vi "Config_Instrument.vi"() -> ()   [LabVIEW 2015]
uses:
  Program Files/National Instruments/LabVIEW 2015/examples/Instrument IO/Serial/support/Serial - Settings.ctl
  <vilib>/Instr/_visa.llb/VISA Configure Serial Port (Instr).vi
  Global_Serial.vi
  <instrlib>/Agilent E363X Series/Agilent E363X Series.lvlib
  <instrlib>/Rohde&Schwarz Spectrum Analyzer/Rohde&Schwarz Spectrum Analyzer.lvlib
panel:
  out "R&S Spec2":refnum<visa-resource-name>
  out "R&S Spec1":refnum<visa-resource-name>
  out "LED_K6":bool
  in  "OK":bool=TRUE
  out "LED_RSSMA":bool
  out "LED_K4":bool
  out "LED_RS S2":bool
  in  "RBW2(HZ)":dbl(knob)=2100000000.0 scale=1000000.0..8000000000.0 scale format="%#_4p"
  in  "Stop Frequency2 (Hz)":dbl(knob)=2100000000.0 scale=1000000.0..8000000000.0 scale format="%#_4p"
  in  "Start Frequency2 (Hz)":dbl(knob)=2100000000.0 scale=1000000.0..8000000000.0 scale format="%#_4p"
  out "LED_RS S1":bool
  in  "RBW(HZ)":dbl(knob)=2100000000.0 scale=1000000.0..8000000000.0 scale format="%#_4p"
  in  "Stop Frequency (Hz)":dbl(knob)=2100000000.0 scale=1000000.0..8000000000.0 scale format="%#_4p"
  in  "Start Frequency (Hz)":dbl(knob)=2100000000.0 scale=1000000.0..8000000000.0 scale format="%#_4p"
  in  "Open XXXXXXXXXXXX":bool
  in  "Open R&S SMA200":bool
  in  "Open R&S Spectrum2":bool
  in  "Open R&S Spectrum1":bool
  in  "Open R&S SMA100":bool
  in  "Open KEYSIGHE E3631#4":bool
  in  "Open KEYSIGHE E3631#6":bool
  in  "SPAN2":dbl(slide)=1000000000.0 scale=1000000.0..8000000000.0 scale format="%#.2p"
  in  "OFFSET2(dBm)":dbl(slide) scale=-20.0..30.0 scale format="%#.2f"
  in  "REF LEVEL2(dBm)":dbl(slide) scale=-20.0..30.0 scale format="%#.2f"
  in  "Center Frequency2(Hz)":dbl(knob)=2100000000.0 scale=1000000.0..8000000000.0 scale format="%#_4p"
  in  "R&S Spectrum2":refnum<visa-resource-name>="COM1"
  in  "SPAN":dbl(slide)=1000000000.0 scale=1000000.0..8000000000.0 scale format="%#.2p"
  in  "OFFSET(dBm)":dbl(slide) scale=-20.0..30.0 scale format="%#.2f"
  in  "REF LEVEL(dBm)":dbl(slide) scale=-20.0..30.0 scale format="%#.2f"
  in  "Center Frequency (Hz)":dbl(knob)=2100000000.0 scale=1000000.0..8000000000.0 scale format="%#_4p"
  in  "R&S Spectrum1":refnum<visa-resource-name>="COM1"
  in  "RF ON":bool
  in  "RF Level(dBm)":dbl(slide) scale=-146.0..18.0 scale format="%#.2f"
  in  "RF Phase":dbl(slide)=154517.79084245834 step=1.0 scale=-360.0..360.0 scale format="%#_6p"
  in  "RF Frequency (Hz)":dbl(knob)=205410.22592152198 scale=1000000.0..3000000000.0 scale format="%#_6p"
  in  "R&S SMA100":refnum<visa-resource-name>="COM1"
  in  "CH2#4":bool
  in  "CH3#4":bool
  in  "CH1#4":bool
  in  "CH2#6":bool
  in  "CH3#6":bool
  in  "CH1#6":bool
  in  "#4最小输入电压(V)":i32=1 min=0 max=6
  in  "#4最大输入电压(V)":i32=2 min=0 max=6
  in  "#6最小输入电压(V)":i32 min=0
  in  "#6最大输入电压(V)":i32=3 min=0
  in  "CC3#4(A)":dbl(slide) scale=0.0..1.0 scale format="%#.2f"
  in  "CC2#4(A)":dbl(slide) scale=0.0..1.0 scale format="%#.2f"
  in  "CC1#4(A)":dbl(slide) scale=0.0..5.0 scale format="%#.2f"
  in  "CV2#4(V)":dbl(slide) scale format="%#.2f"
  in  "CV1#4(V)":dbl(slide) scale=0.0..25.0 scale format="%#.2f"
  in  "CV3#4(V)":dbl(slide) scale=0.0..6.0 scale format="%#.2f"
  out "Instrument Driver Revision 2":string="*IDN?"
  in  "CC3#6(A)":dbl(slide) scale=0.0..1.0 scale format="%#.2f"
  in  "CC2#6(A)":dbl(slide) scale=0.0..1.0 scale format="%#.2f"
  in  "CC1#6(A)":dbl(slide) scale=0.0..5.0 scale format="%#.2f"
  in  "CV2#6(V)":dbl(slide) scale format="%#.2f"
  in  "CV1#6(V)":dbl(slide) scale=0.0..25.0 scale format="%#.2f"
  in  "CV3#6(V)":dbl(slide) scale=0.0..6.0 scale format="%#.2f"
  out "Instrument Driver Revision":string="*IDN?"
  in  "KeysightE363x_#4":refnum<visa-resource-name>="COM1"
  in  "KeysightE363x_#6":refnum<visa-resource-name>="COM1"
  in  "stop":bool
  in  "error in (no error)":errorcluster
  in  "SerialON":bool
  in  "Serial Settings":T1={"baud rate"=9600, "data bits"=8, "parity"=enum."None", "stop bits"=10, "flow control"=0} {"flow control" items=["None"=0, "XON/XOFF"=1, "RTS/CTS"=2, "DTR/DSR"=4]; "stop bits" items=["1.0"=10, "1.5"=15, "2.0"=20]; "data bits" min=5 max=8 step=1; "baud rate" items=["75"=75, "110"=110, "134"=134, "150"=150, "300"=300, "600"=600, "1200"=1200, "1800"=1800, "2400"=2400, "4800"=4800, "7200"=7200, "9600"=9600, "14400"=14400, "19200"=19200, "28800"=28800, "38400"=38400, "56000"=56000, "57600"=57600, "115200"=115200, "128000"=128000, "230400"=230400]}
  in  "Serial Port":refnum<visa-resource-name>="COM1"
  # "缺省信号源"
  # "缺省信号源"
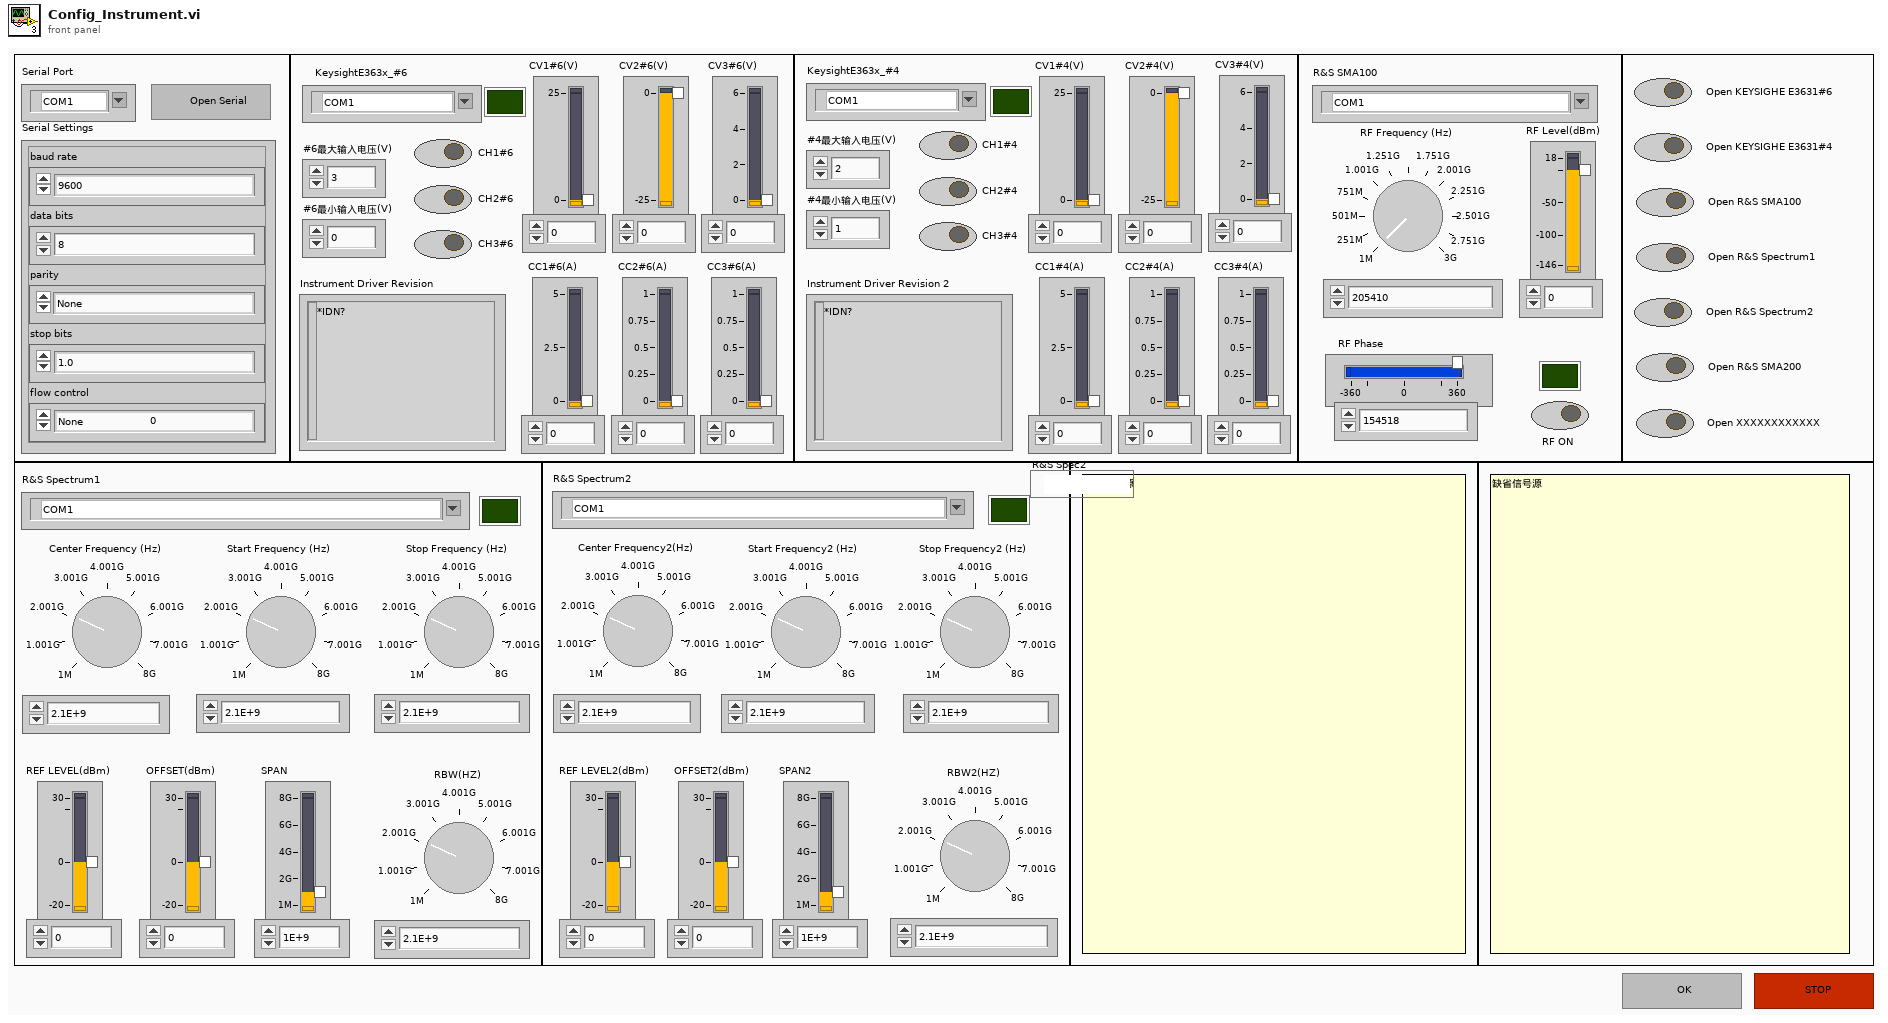
[diagram p1: front panel]
types:
  T1 = typedef "Serial - Settings.ctl" = cluster{"baud rate":u32, "data bits":u16, "parity":enum16{"None", "Odd", "Even", "Mark", "Space"}, "stop bits":u16, "flow control":u16}
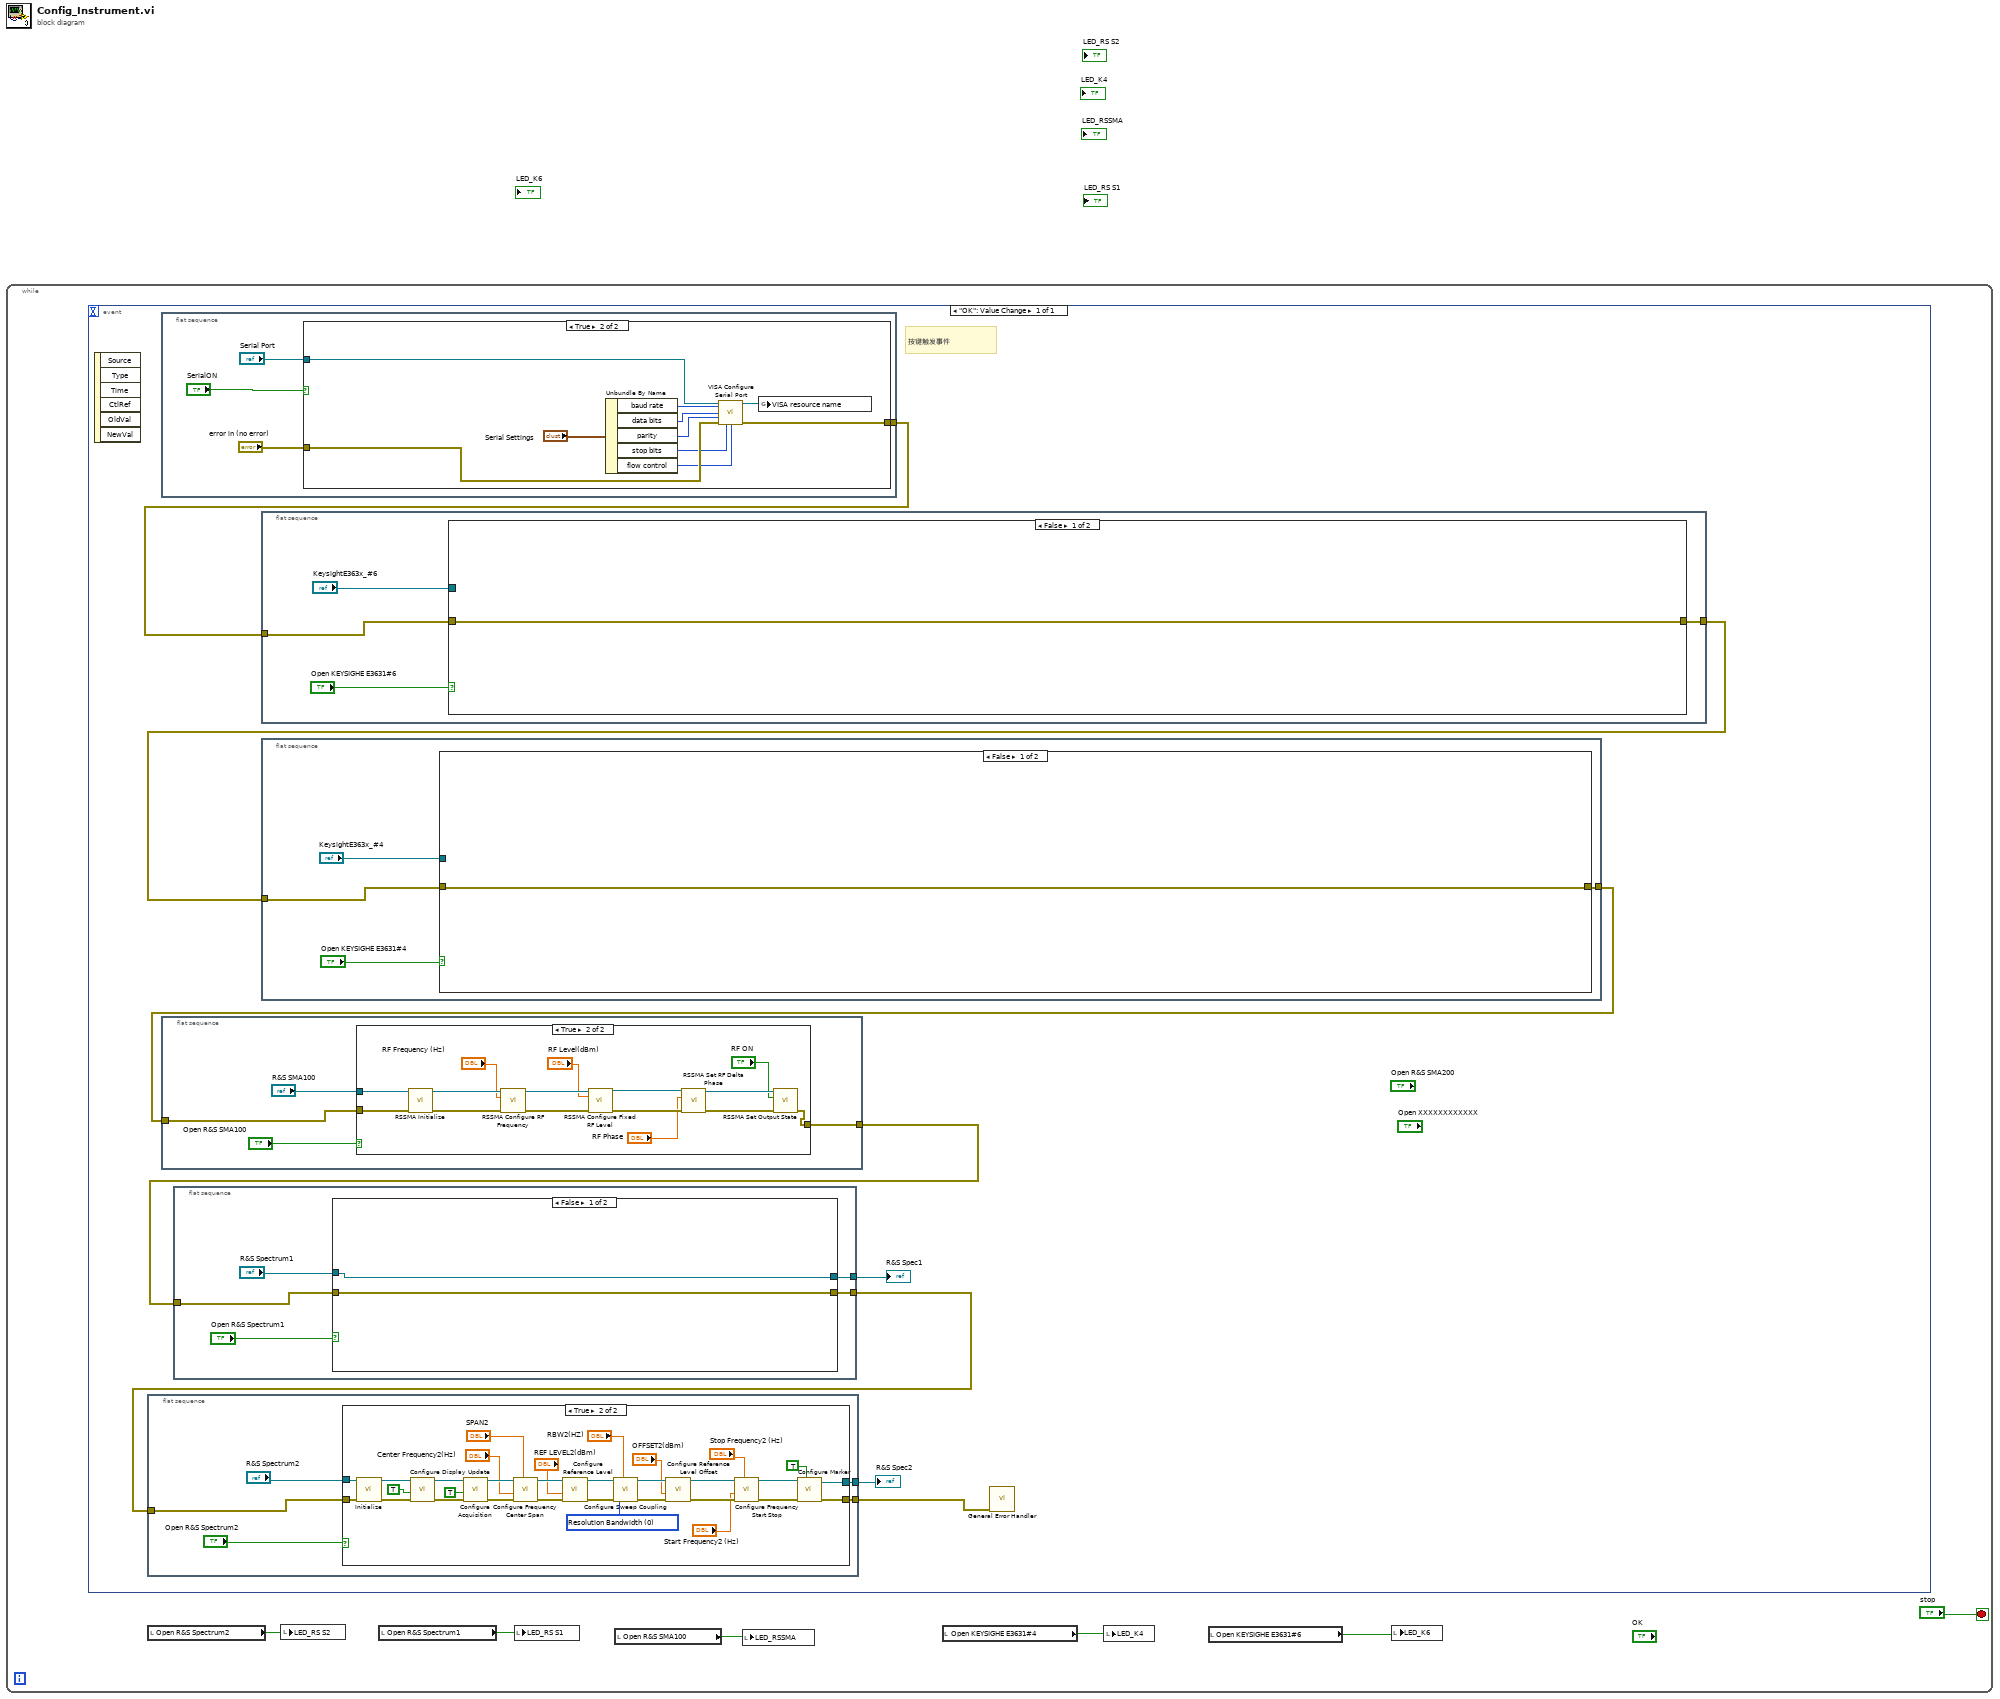
[diagram p0: block diagram]
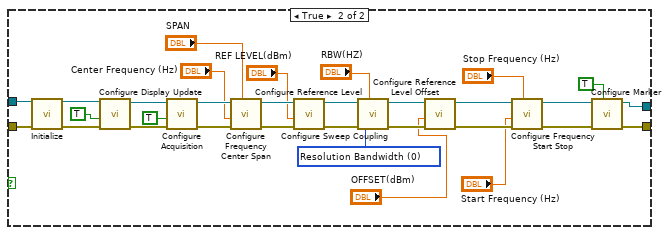
[diagram p3: hidden frame]
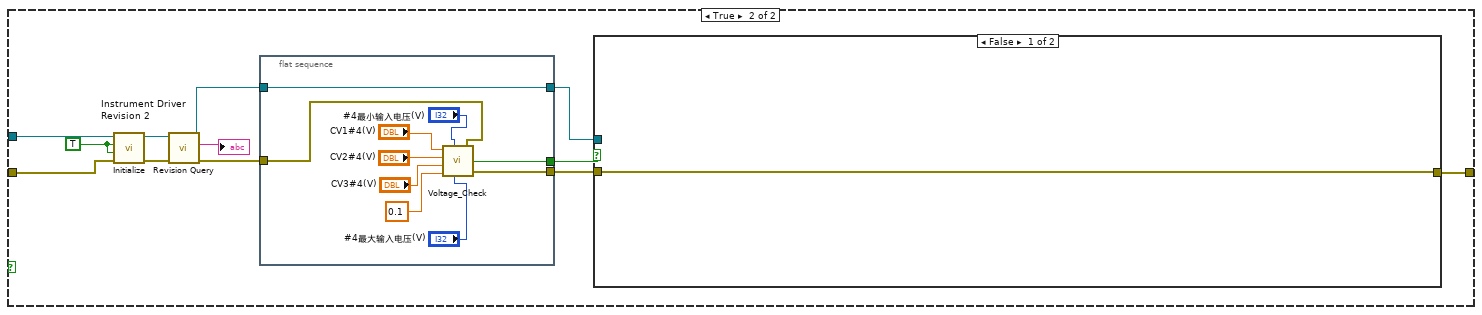
[diagram p5: hidden frame]
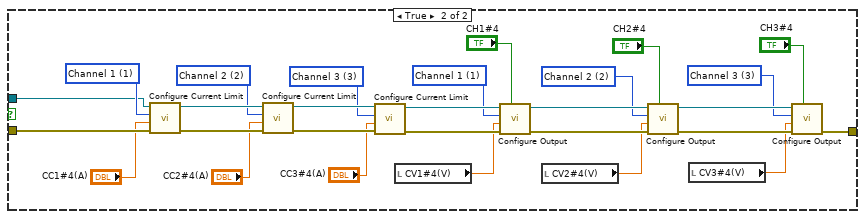
[diagram p6: hidden frame]
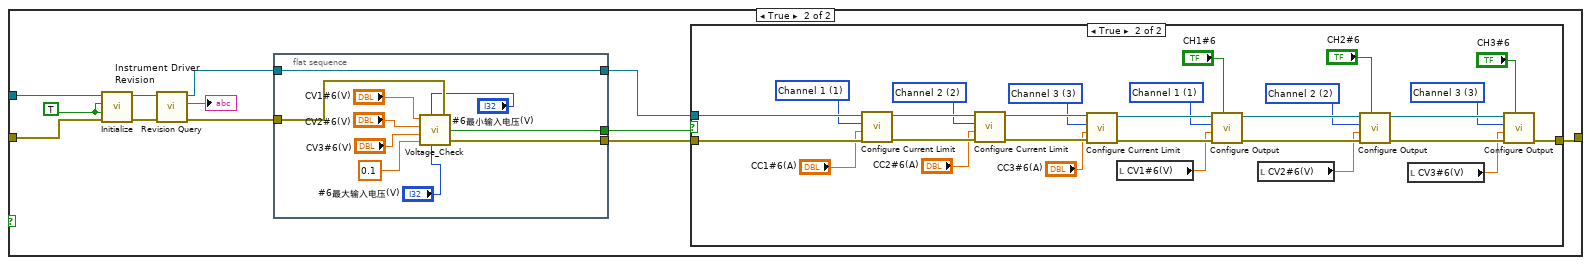
[diagram p7: hidden frame]
diagram:
  n1 = while {
    stop <- "stop" stop-if-true
    n2 = event shown="[0] \"OK\": Value Change" {
      selector: _ -> [_]
      dyn-events: _ -> [_]
      timeout: _ -> [_]
      event "OK": Value Change {
        # "按键触发事件"
        n3 = event-data() -> ()  [unwired: 1 in, 6 out]
        n4 = flat-sequence {
          tunnel: w10 -> [w17]
          tunnel: [w16] -> w9
          tunnel: [w15] -> w7
          frame #0 {
            n5 = case shown="True" "Open R&S Spectrum2" {
              tunnel: w17 -> [w21 w36]
              tunnel: "R&S Spectrum2" -> [w20 w27]
              tunnel: [w21 w23] -> w16
              tunnel: [w20 w22] -> w15
              frame False {
              }
              frame True {
                w37 = 0 items=["Resolution Bandwidth", "Video Bandwidth", "Sweep Time"] ("Sweep Coupling (Resolution Bandwidth)")
                n6 = call <instrlib>:"Initialize.vi"("VISA resource name"=w27, "error in (no error)"=w36) -> ("VISA resource name out"=w50:refnum<visa-resource-name>, "error out"=w51:errorcluster)  [unwired: 12 in]
                n7 = call <instrlib>:"Configure Display Update.vi"("error in (no error)"=w51, "Display In Remote (F: Off)"=TRUE, "VISA resource name"=w50) -> ("error out"=w49:errorcluster, "VISA resource name out"=w48:refnum<visa-resource-name>)  [unwired: 7 in]
                n8 = call <instrlib>:"Configure Acquisition.vi"("error in (no error)"=w49, "Sweep Mode Continuous (F: Off)"=TRUE, "VISA resource name"=w48) -> ("error out"=w46:errorcluster, "VISA resource name out"=w45:refnum<visa-resource-name>)  [unwired: 7 in]
                n9 = call <instrlib>:"Configure Frequency Center Span.vi"("Span (0.0)"="SPAN2", "error in (no error)"=w46, "Center Frequency (0.0)"="Center Frequency2(Hz)", "VISA resource name"=w45) -> ("error out"=w44:errorcluster, "VISA resource name out"=w43:refnum<visa-resource-name>)  [unwired: 6 in]
                n10 = call <instrlib>:"Configure Reference Level.vi"("error in (no error)"=w44, "Reference Level (-20.0)"="REF LEVEL2(dBm)", "VISA resource name"=w43) -> ("error out"=w42:errorcluster, "VISA resource name out"=w41:refnum<visa-resource-name>)  [unwired: 7 in]
                n11 = call <instrlib>:"Configure Sweep Coupling.vi"("Coupling Value (0.0)"="RBW2(HZ)", "error in (no error)"=w42, "Sweep Coupling (Resolution Bandwidth)"=w37, "VISA resource name"=w41) -> ("error out"=w40:errorcluster, "VISA resource name out"=w39:refnum<visa-resource-name>)  [unwired: 6 in]
                n12 = call <instrlib>:"Configure Reference Level Offset.vi"("error in (no error)"=w40, "Reference Level Offset (0.0)"="OFFSET2(dBm)", "VISA resource name"=w39) -> ("error out"=w35:errorcluster, "VISA resource name out"=w34:refnum<visa-resource-name>)  [unwired: 7 in]
                n13 = call <instrlib>:"Configure Frequency Start Stop.vi"("Stop Frequency (0.0)"="Stop Frequency2 (Hz)", "error in (no error)"=w35, "Start Frequency (0.0)"="Start Frequency2 (Hz)", "VISA resource name"=w34) -> ("error out"=w33:errorcluster, "VISA resource name out"=w32:refnum<visa-resource-name>)  [unwired: 6 in]
                n14 = call <instrlib>:"Configure Marker.vi"("Marker State (F: Off)"=TRUE, "error in (no error)"=w33, "VISA resource name"=w32) -> ("error out"=w23:errorcluster, "VISA resource name out"=w22:refnum<visa-resource-name>)  [unwired: 7 in]
              }
            }
          }
        }
        n15 = flat-sequence {
          tunnel: [w223] -> w14
          frame #0 {
            n16 = case shown="True" "SerialON" {
              tunnel: "Serial Port" -> [_ w237]
              tunnel: "error in (no error)" -> [w227 w236]
              tunnel: [w227 w229] -> w223
              frame False {
              }
              frame True {
                n17 = Unbundle By Name("Serial Settings") -> ("baud rate"=w231:u32, "data bits"=w232:u16, "parity"=w233:enum16{"None", "Odd", "Even", "Mark", "Space"}, "stop bits"=w234:u16, "flow control"=w235:u16)
                n18 = call-poly "VISA Configure Serial Port"("VISA resource name"=w237, "baud rate (9600)"=w231, "data bits (8)"=w232, "parity (0:none)"=w233, "error in (no error)"=w236, "stop bits (10: 1 bit)"=w234, "flow control (0:none)"=w235) -> ("VISA resource name out"=w228:refnum<visa-resource-name>, "error out"=w229:errorcluster)  [unwired: 7 in]
                n19 = global write "Global_Serial.vi" "VISA resource name"(w228) -> ()
              }
            }
          }
        }
        n20 = flat-sequence {
          tunnel: w12 -> [w92]
          tunnel: [w91] -> w11
          frame #0 {
            n21 = case shown="True" "Open R&S SMA100" {
              tunnel: "R&S SMA100" -> [_ w102]
              tunnel: w92 -> [w95 w101]
              tunnel: [w95 w96] -> w91
              frame False {
              }
              frame True {
                n22 = call <instrlib>:"RSSMA Initialize.vi"("error in (no error)"=w101, "Resource Name (GPIB::28)"=w102) -> ("error out"=w110:errorcluster, "dup VISA session"=w109:refnum<visa-resource-name>)  [unwired: 8 in]
                n23 = call <instrlib>:"RSSMA Configure RF Frequency.vi"("error in (no error)"=w110, "Frequency (1.0e9 Hz)"="RF Frequency (Hz)", "VISA session"=w109) -> ("error out"=w108:errorcluster, "dup VISA session"=w107:refnum<visa-resource-name>)  [unwired: 7 in]
                n24 = call <instrlib>:"RSSMA Configure Fixed RF Level.vi"("VISA session"=w107, "Amplitude (-30.0 dBm)"="RF Level(dBm)", "error in (no error)"=w108) -> ("dup VISA session"=w105:refnum<visa-resource-name>, "error out"=w106:errorcluster)  [unwired: 11 in]
                n25 = call <instrlib>:"RSSMA Set RF Delta Phase.vi"("error in (no error)"=w106, "Delta Phase (0.0)"="RF Phase", "VISA session"=w105) -> ("error out"=w104:errorcluster, "dup VISA session"=w103:refnum<visa-resource-name>)  [unwired: 7 in]
                n26 = call <instrlib>:"RSSMA Set Output State.vi"("error in (no error)"=w104, "RF Output State (F: Off)"="RF ON", "VISA session"=w103) -> ("error out"=w96:errorcluster)  [unwired: 7 in, 1 out]
              }
            }
          }
        }
        n27 = flat-sequence {
          tunnel: w11 -> [w55]
          tunnel: [w54] -> w10
          tunnel: [w53] -> w8
          frame #0 {
            n28 = case shown="False" "Open R&S Spectrum1" {
              tunnel: w55 -> [w59 w74]
              tunnel: "R&S Spectrum1" -> [w58 w69]
              tunnel: [w59 w61] -> w54
              tunnel: [w58 w60] -> w53
              frame False {
              }
              frame True {
                w75 = 0 items=["Resolution Bandwidth", "Video Bandwidth", "Sweep Time"] ("Sweep Coupling (Resolution Bandwidth)")
                n29 = call <instrlib>:"Initialize.vi"("VISA resource name"=w69, "error in (no error)"=w74) -> ("VISA resource name out"=w88:refnum<visa-resource-name>, "error out"=w89:errorcluster)  [unwired: 12 in]
                n30 = call <instrlib>:"Configure Display Update.vi"("error in (no error)"=w89, "Display In Remote (F: Off)"=TRUE, "VISA resource name"=w88) -> ("error out"=w87:errorcluster, "VISA resource name out"=w86:refnum<visa-resource-name>)  [unwired: 7 in]
                n31 = call <instrlib>:"Configure Acquisition.vi"("error in (no error)"=w87, "Sweep Mode Continuous (F: Off)"=TRUE, "VISA resource name"=w86) -> ("error out"=w84:errorcluster, "VISA resource name out"=w83:refnum<visa-resource-name>)  [unwired: 7 in]
                n32 = call <instrlib>:"Configure Frequency Center Span.vi"("Span (0.0)"="SPAN", "error in (no error)"=w84, "Center Frequency (0.0)"="Center Frequency (Hz)", "VISA resource name"=w83) -> ("error out"=w82:errorcluster, "VISA resource name out"=w81:refnum<visa-resource-name>)  [unwired: 6 in]
                n33 = call <instrlib>:"Configure Reference Level.vi"("error in (no error)"=w82, "Reference Level (-20.0)"="REF LEVEL(dBm)", "VISA resource name"=w81) -> ("error out"=w80:errorcluster, "VISA resource name out"=w79:refnum<visa-resource-name>)  [unwired: 7 in]
                n34 = call <instrlib>:"Configure Sweep Coupling.vi"("Coupling Value (0.0)"="RBW(HZ)", "error in (no error)"=w80, "Sweep Coupling (Resolution Bandwidth)"=w75, "VISA resource name"=w79) -> ("error out"=w78:errorcluster, "VISA resource name out"=w77:refnum<visa-resource-name>)  [unwired: 6 in]
                n35 = call <instrlib>:"Configure Reference Level Offset.vi"("error in (no error)"=w78, "Reference Level Offset (0.0)"="OFFSET(dBm)", "VISA resource name"=w77) -> ("error out"=w73:errorcluster, "VISA resource name out"=w72:refnum<visa-resource-name>)  [unwired: 7 in]
                n36 = call <instrlib>:"Configure Frequency Start Stop.vi"("Stop Frequency (0.0)"="Stop Frequency (Hz)", "error in (no error)"=w73, "Start Frequency (0.0)"="Start Frequency (Hz)", "VISA resource name"=w72) -> ("error out"=w71:errorcluster, "VISA resource name out"=w70:refnum<visa-resource-name>)  [unwired: 6 in]
                n37 = call <instrlib>:"Configure Marker.vi"("Marker State (F: Off)"=TRUE, "error in (no error)"=w71, "VISA resource name"=w70) -> ("error out"=w61:errorcluster, "VISA resource name out"=w60:refnum<visa-resource-name>)  [unwired: 7 in]
              }
            }
          }
        }
        n38 = flat-sequence {
          tunnel: w14 -> [w168]
          tunnel: [w167] -> w13
          frame #0 {
            n39 = case shown="False" "Open KEYSIGHE E3631#6" {
              tunnel: "KeysightE363x_#6" -> [_ w183]
              tunnel: w168 -> [w171 w174]
              tunnel: [w171 w172] -> w167
              frame False {
              }
              frame True {
                w173 = TRUE ("Reset? (T: Yes)")
                n40 = call <instrlib>:"Initialize.vi"("error in (no error)"=w174, "Reset? (T: Yes)"=w173, "ID Query? (T: Yes)"=w173, "VISA resource name"=w183) -> ("error out"=w182:errorcluster, "VISA resource name out"=w181:refnum<visa-resource-name>)  [unwired: 6 in]
                n41 = call <instrlib>:"Revision Query.vi"("error in (no error)"=w182, "VISA resource name"=w181) -> ("error out"=w179:errorcluster, "Instrument Driver Revision"=→"Instrument Driver Revision":string, "VISA resource name out"=w177:refnum<visa-resource-name>)  [unwired: 6 in, 1 out]
                n42 = flat-sequence {
                  tunnel: w179 -> [w222]
                  tunnel: [w221] -> w178
                  tunnel: w177 -> [w221]
                  tunnel: [w220] -> w176
                  tunnel: [w216] -> w175
                  frame #0 {
                    n43 = call "Voltage_Check.vi"("channel1"="CV1#6(V)", "limitmin"="#6最小输入电压(V)", "channel2"="CV2#6(V)", "channel3"="CV3#6(V)", "limitmax"="#6最大输入电压(V)", "channel4"=0.1 ("y"), "error in (no error) 2"=w222) -> ("state"=w216:bool, "error out 2"=w220:errorcluster)
                  }
                }
                n44 = case shown="True" w175 {
                  tunnel: w178 -> [_ w212]
                  tunnel: w176 -> [w184 w211]
                  tunnel: [w184 w185] -> w172
                  frame False {
                  }
                  frame True {
                    w195 = 3 items=["Channel 1"=1, "Channel 2"=2, "Channel 3"=3] ("Channel (1: Channel 1)")
                    w196 = 2 items=["Channel 1"=1, "Channel 2"=2, "Channel 3"=3] ("Channel (1: Channel 1)")
                    w197 = 1 items=["Channel 1"=1, "Channel 2"=2, "Channel 3"=3] ("Channel (1: Channel 1)")
                    w204 = 3 items=["Channel 1"=1, "Channel 2"=2, "Channel 3"=3] ("Channel (1: Channel 1)")
                    w205 = 2 items=["Channel 1"=1, "Channel 2"=2, "Channel 3"=3] ("Channel (1: Channel 1)")
                    w208 = 1 items=["Channel 1"=1, "Channel 2"=2, "Channel 3"=3] ("Channel (1: Channel 1)")
                    n45 = call <instrlib>:"Configure Current Limit.vi"("error in (no error)"=w211, "Current Limit (0.0 A)"="CC1#6(A)", "Channel (1: Channel 1)"=w208, "VISA resource name"=w212) -> ("error out"=w210:errorcluster, "VISA resource name out"=w207:refnum<visa-resource-name>)  [unwired: 6 in]
                    n46 = call <instrlib>:"Configure Current Limit.vi"("error in (no error)"=w210, "Current Limit (0.0 A)"="CC2#6(A)", "Channel (1: Channel 1)"=w205, "VISA resource name"=w207) -> ("error out"=w209:errorcluster, "VISA resource name out"=w206:refnum<visa-resource-name>)  [unwired: 6 in]
                    n47 = call <instrlib>:"Configure Current Limit.vi"("error in (no error)"=w209, "Current Limit (0.0 A)"="CC3#6(A)", "Channel (1: Channel 1)"=w204, "VISA resource name"=w206) -> ("error out"=w203:errorcluster, "VISA resource name out"=w202:refnum<visa-resource-name>)  [unwired: 6 in]
                    n48 = local read "CV1#6(V)"() -> (w191:dbl)
                    n49 = call <instrlib>:"Configure Output.vi"("Enable Output (T: Enable)"="CH1#6", "error in (no error)"=w203, "Voltage Level (0.0 V)"=w191, "Channel (1: Channel 1)"=w197, "VISA resource name"=w202) -> ("error out"=w201:errorcluster, "VISA resource name out"=w200:refnum<visa-resource-name>)  [unwired: 5 in]
                    n50 = local read "CV2#6(V)"() -> (w190:dbl)
                    n51 = call <instrlib>:"Configure Output.vi"("Enable Output (T: Enable)"="CH2#6", "error in (no error)"=w201, "Voltage Level (0.0 V)"=w190, "Channel (1: Channel 1)"=w196, "VISA resource name"=w200) -> ("error out"=w199:errorcluster, "VISA resource name out"=w198:refnum<visa-resource-name>)  [unwired: 5 in]
                    n52 = local read "CV3#6(V)"() -> (w189:dbl)
                    n53 = call <instrlib>:"Configure Output.vi"("Enable Output (T: Enable)"="CH3#6", "error in (no error)"=w199, "Voltage Level (0.0 V)"=w189, "Channel (1: Channel 1)"=w195, "VISA resource name"=w198) -> ("error out"=w185:errorcluster)  [unwired: 5 in, 1 out]
                  }
                }
              }
            }
          }
        }
        n54 = flat-sequence {
          tunnel: w13 -> [w112]
          tunnel: [w111] -> w12
          frame #0 {
            n55 = case shown="False" "Open KEYSIGHE E3631#4" {
              tunnel: "KeysightE363x_#4" -> [_ w127]
              tunnel: w112 -> [w115 w125]
              tunnel: [w115 w116] -> w111
              frame False {
              }
              frame True {
                w126 = TRUE ("Reset? (T: Yes)")
                n56 = call <instrlib>:"Initialize.vi"("error in (no error)"=w125, "Reset? (T: Yes)"=w126, "ID Query? (T: Yes)"=w126, "VISA resource name"=w127) -> ("error out"=w123:errorcluster, "VISA resource name out"=w124:refnum<visa-resource-name>)  [unwired: 6 in]
                n57 = call <instrlib>:"Revision Query.vi"("error in (no error)"=w123, "VISA resource name"=w124) -> ("error out"=w121:errorcluster, "Instrument Driver Revision"=→"Instrument Driver Revision 2":string, "VISA resource name out"=w117:refnum<visa-resource-name>)  [unwired: 6 in, 1 out]
                n58 = flat-sequence {
                  tunnel: w121 -> [w131]
                  tunnel: [w130] -> w120
                  tunnel: [w129] -> w119
                  tunnel: [w128] -> w118
                  tunnel: w117 -> [w128]
                  frame #0 {
                    n59 = call "Voltage_Check.vi"("channel1"="CV1#4(V)", "limitmin"="#4最小输入电压(V)", "channel2"="CV2#4(V)", "channel3"="CV3#4(V)", "limitmax"="#4最大输入电压(V)", "channel4"=0.1, "error in (no error) 2"=w131) -> ("state"=w129:bool, "error out 2"=w130:errorcluster)
                  }
                }
                n60 = case shown="False" w119 {
                  tunnel: w120 -> [w138 w166]
                  tunnel: w118 -> [_ w140]
                  tunnel: [w138 w139] -> w116
                  frame False {
                  }
                  frame True {
                    w147 = 3 items=["Channel 1"=1, "Channel 2"=2, "Channel 3"=3] ("Channel (1: Channel 1)")
                    w148 = 2 items=["Channel 1"=1, "Channel 2"=2, "Channel 3"=3] ("Channel (1: Channel 1)")
                    w149 = 1 items=["Channel 1"=1, "Channel 2"=2, "Channel 3"=3] ("Channel (1: Channel 1)")
                    w150 = 3 items=["Channel 1"=1, "Channel 2"=2, "Channel 3"=3] ("Channel (1: Channel 1)")
                    w151 = 2 items=["Channel 1"=1, "Channel 2"=2, "Channel 3"=3] ("Channel (1: Channel 1)")
                    w152 = 1 items=["Channel 1"=1, "Channel 2"=2, "Channel 3"=3] ("Channel (1: Channel 1)")
                    n61 = call <instrlib>:"Configure Current Limit.vi"("error in (no error)"=w166, "Current Limit (0.0 A)"="CC1#4(A)", "Channel (1: Channel 1)"=w152, "VISA resource name"=w140) -> ("error out"=w165:errorcluster, "VISA resource name out"=w160:refnum<visa-resource-name>)  [unwired: 6 in]
                    n62 = call <instrlib>:"Configure Current Limit.vi"("error in (no error)"=w165, "Current Limit (0.0 A)"="CC2#4(A)", "Channel (1: Channel 1)"=w151, "VISA resource name"=w160) -> ("error out"=w164:errorcluster, "VISA resource name out"=w159:refnum<visa-resource-name>)  [unwired: 6 in]
                    n63 = call <instrlib>:"Configure Current Limit.vi"("error in (no error)"=w164, "Current Limit (0.0 A)"="CC3#4(A)", "Channel (1: Channel 1)"=w150, "VISA resource name"=w159) -> ("error out"=w163:errorcluster, "VISA resource name out"=w158:refnum<visa-resource-name>)  [unwired: 6 in]
                    n64 = local read "CV1#4(V)"() -> (w143:dbl)
                    n65 = call <instrlib>:"Configure Output.vi"("Enable Output (T: Enable)"="CH1#4", "error in (no error)"=w163, "Voltage Level (0.0 V)"=w143, "Channel (1: Channel 1)"=w149, "VISA resource name"=w158) -> ("error out"=w162:errorcluster, "VISA resource name out"=w157:refnum<visa-resource-name>)  [unwired: 5 in]
                    n66 = local read "CV2#4(V)"() -> (w142:dbl)
                    n67 = call <instrlib>:"Configure Output.vi"("Enable Output (T: Enable)"="CH2#4", "error in (no error)"=w162, "Voltage Level (0.0 V)"=w142, "Channel (1: Channel 1)"=w148, "VISA resource name"=w157) -> ("error out"=w161:errorcluster, "VISA resource name out"=w156:refnum<visa-resource-name>)  [unwired: 5 in]
                    n68 = local read "CV3#4(V)"() -> (w141:dbl)
                    n69 = call <instrlib>:"Configure Output.vi"("Enable Output (T: Enable)"="CH3#4", "error in (no error)"=w161, "Voltage Level (0.0 V)"=w141, "Channel (1: Channel 1)"=w147, "VISA resource name"=w156) -> ("error out"=w139:errorcluster)  [unwired: 5 in, 1 out]
                  }
                }
              }
            }
          }
        }
        n70 = call <vilib>:"General Error Handler.vi"("error in (no error)"=w9) -> ()  [unwired: 10 in, 5 out]
        "R&S Spec1" <- w8
        "R&S Spec2" <- w7
      }
    }
    n71 = local read "Open R&S Spectrum2"() -> (w4:bool)
    n72 = local write "LED_RS S2"(w4) -> ()
    n73 = local read "Open R&S Spectrum1"() -> (w3:bool)
    n74 = local write "LED_RS S1"(w3) -> ()
    n75 = local read "Open R&S SMA100"() -> (w2:bool)
    n76 = local write "LED_RSSMA"(w2) -> ()
    n77 = local read "Open KEYSIGHE E3631#4"() -> (w1:bool)
    n78 = local write "LED_K4"(w1) -> ()
    n79 = local read "Open KEYSIGHE E3631#6"() -> (w5:bool)
    n80 = local write "LED_K6"(w5) -> ()
  }
